vi "Check Initialization Status.vi"(0 "UART Driver in":refnum<class "UART Driver.lvclass">, 11 "error in":errorcluster) -> (4 "UART Driver out":refnum<class "UART Driver.lvclass">, 15 "error out":errorcluster)   [LabVIEW 2012, in "UART_Host_Driver.lvlib" / "UART Driver.lvclass"]
doc: "Check to make sure the UART FPGA personality has completed the required startup operations."
uses:
  UART Driver.lvclass
  Typedefs/FPGA VI Reference.ctl
  UART Driver.lvclass/UART Driver.ctl
  <vilib>/Utility/error.llb/Error Cluster From Error Code.vi
  <vilib>/rvi/errors/niLvFpgaAdjustHostInterfaceError.vi
  <vilib>/rvi/interface/nirviReadWriteControl/nirviReadWriteControl.xnode
  <vilib>/ErrorRing/Error Ring.xnode
  UART_Host_Driver.lvlib
  NiFpgaLv.dll
  <vilib>/rvi/interface/Simulation/niFpgaSimulationCallBeginRW.vi
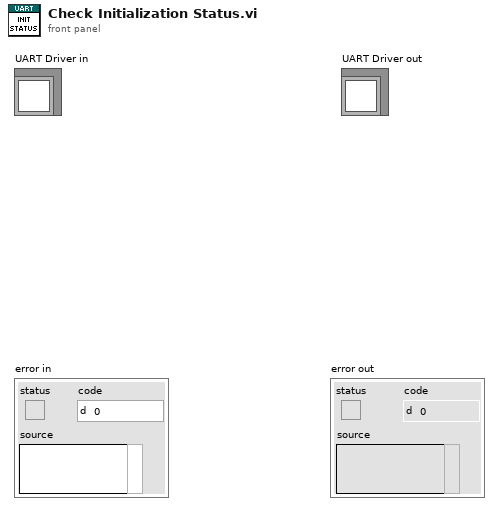
[diagram p1: front panel]
types:
  T1 = typedef "UART_Host_Driver.lvlib/FPGA VI Reference.ctl" = refnum<k20>
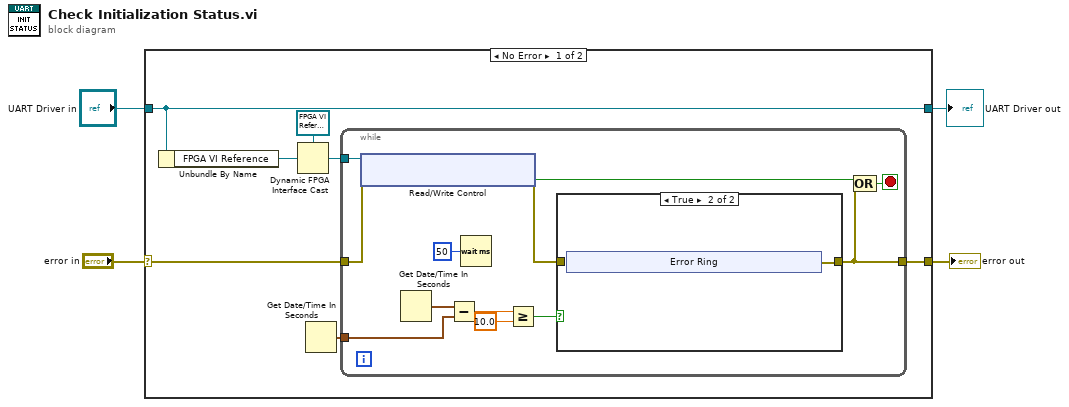
[diagram p0: block diagram]
diagram:
  n1 = case shown="No Error" "error in" {
    selector: "error in" -> [w8 w31]
    tunnel: [w5 w31] -> w3
    tunnel: [w7 w30] -> w2
    tunnel: "UART Driver in" -> [w7 w30]
    frame No Error {
      n2 = Unbundle By Name(w7) -> ("FPGA VI Reference"=w11:refnum<k20>)
      n3 = Dynamic FPGA Interface Cast(Session In=T1 refnum ("FPGA VI Reference"), Type=w11) -> (Session Out=w9:T1)
      n4 = Get Date/Time In Seconds() -> (seconds since 1Jan1904=w6:timestamp)
      n5 = while {
        tunnel: w9 -> [w23]
        tunnel: w8 -> [w22]
        tunnel: w6 -> [w20]
        tunnel: [w13] -> w5
        stop <- w14 stop-if-true
        n6 = xnode "Read/Write Control"("FPGA VI Reference In"=w23, "error in"=w22) -> ("error out"=w15:errorcluster, "FPGA Initialization Complete?"=w18:bool)  [unwired: 1 out]
        n7 = Get Date/Time In Seconds() -> (seconds since 1Jan1904=w21:timestamp)
        n8 = Subtract(x=w21, y=w20) -> (x-y=w19:dbl)
        n9 = Wait (ms)(milliseconds to wait=u32 50) -> ()  [unwired: 1 out]
        n10 = Greater Or Equal?(x=w19, y=10.0) -> (x >= y?=w16:bool)
        n11 = case shown="True" w16 {
          tunnel: w15 -> [w24 _]
          tunnel: [w24 w25] -> w13
          frame False {
          }
          frame True {
            n12 = xnode "Error Ring"() -> ("error out"=w25:errorcluster)
          }
        }
        n13 = Compound Arithmetic op=OR(w18, w13) -> (w14:bool)
      }
    }
    frame Error {
    }
  }
  "error out" <- w3
  "UART Driver out" <- w2
